vi "deploy callback.vi"(8 "error in":errorcluster, 9 "OS":T1, 10 "IP Address":string, 11 "CVT Engine Editor in":refnum<class "CVT Engine Editor.lvclass">) -> (0 "error out":errorcluster, 3 "CVT Engine Editor out":refnum<class "CVT Engine Editor.lvclass">)   [LabVIEW 2013, in "CVT Engine Editor.lvclass"]
uses:
  CVT Engine Editor.lvclass
  <vilib>/NI/Tag Bus Module Framework/root configuration/Target Types.ctl
  <vilib>/NI/Tag Bus Data Framework/Configuration Editor/Classes/Engine Parent/Engine Parent Editor Node.lvclass
  <vilib>/NI/Tag Bus Module Framework/root configuration/TBM configuration.lvclass
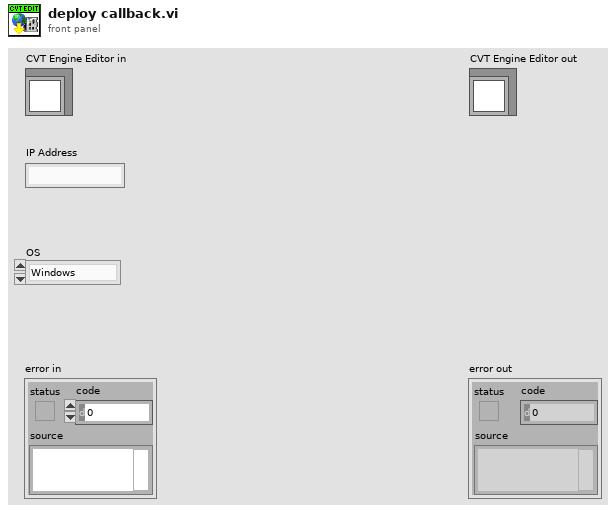
[diagram p1: front panel]
types:
  T1 = typedef "TBM configuration.lvclass/Target Types.ctl" = enum16{"Windows", "Mac", "Linux", "Linux RT ARM", "VxWorks", "Pharlap", "Other", "Linux RT x64"}
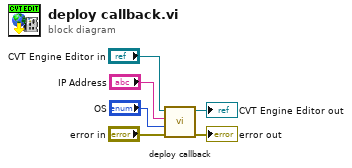
[diagram p0: block diagram]
diagram:
  n1 = call-parent "deploy callback.vi"("error in"="error in", "Target Types"="OS", "IP Address"="IP Address", "TBM Configuration Node in"="CVT Engine Editor in") -> ("error out"=→"error out":errorcluster, "TBM Configuration Node out"=→"CVT Engine Editor out":refnum<class "CVT Engine Editor.lvclass">)  [unwired: 6 in]
